vi "test resources list.vi"(8 "error in (no error)":errorcluster) -> (0 "error out":errorcluster, 3 "body":string)   [LabVIEW 2020, in "MCP Server tests.lvlib"]
uses:
  MCP Server tests.lvlib
  <vilib>/JDP Science/JSONtext/Next JSON Value.vi
  <vilib>/JDP Science/JSONtext/String Subset.vi
  <vilib>/JDP Science/JSONtext/Parsing/Advance past next JSON Value (inlined COPY).vi
  <vilib>/JDP Science/JSONtext/Parsing/Advance past whitespace.vi
  <vilib>/JDP Science/JSONtext/Parsing/Advance past String.vi
  <vilib>/JDP Science/JSONtext/Parsing/Advance past Number.vi
  <vilib>/JDP Science/JSONtext/Parsing/Advance past Line Ending.vi
  <vilib>/JDP Science/JSONtext/Parsing/Parse Full Path or Item Name.vi
  <vilib>/JDP Science/JSONtext/Parsing/Advance past Array.vi
  <vilib>/JDP Science/JSONtext/Parsing/Advance past Object.vi
  <vilib>/JDP Science/JSONtext/support/Error Cluster From Code.vi
  <vilib>/JDP Science/JSONtext/Offset/Find Item Locations by Path.vi
  <vilib>/addons/_JKI Toolkits/Caraya/classes/Test/Test.lvclass
  <vilib>/addons/_JKI Toolkits/Caraya/classes/Assert/Assert.lvclass
  <vilib>/JDP Science/JSONtext/JSONtext.lvlib
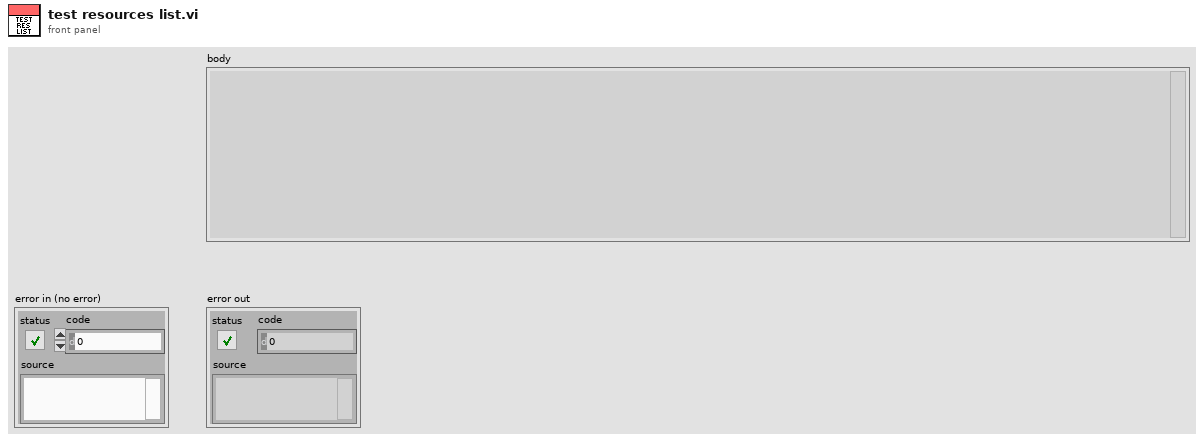
[diagram p1: front panel]
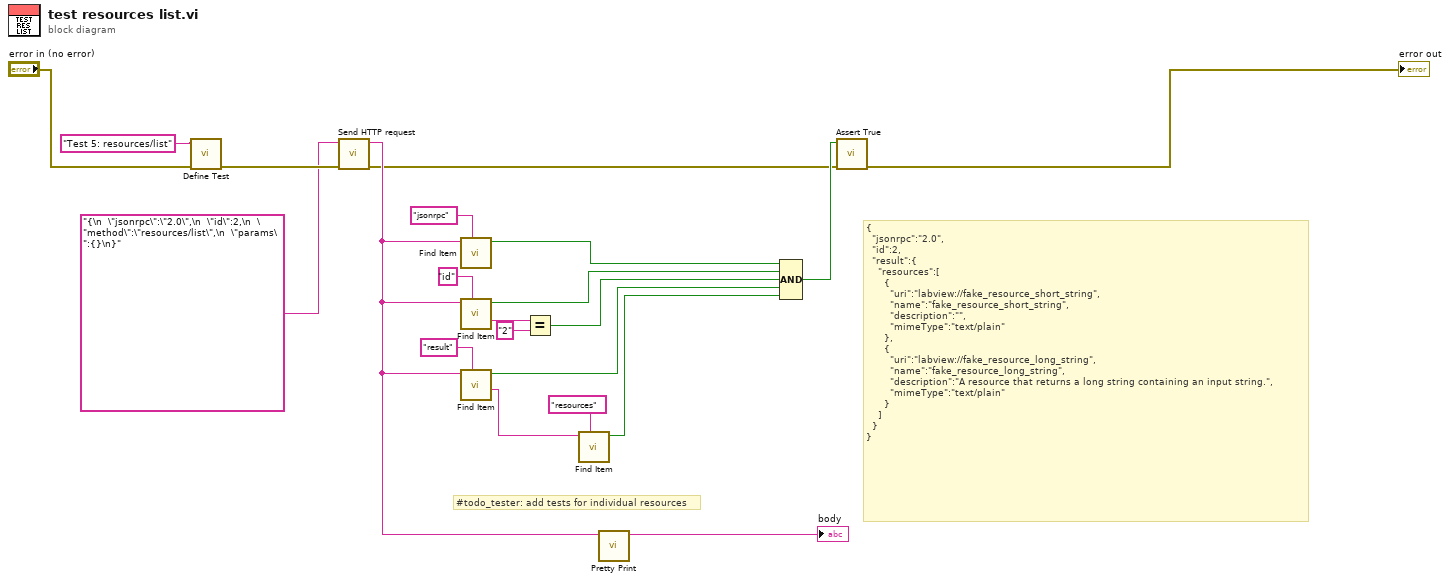
[diagram p0: block diagram]
diagram:
  # "#todo_tester: add tests for individual resources"
  # "{\n  \"jsonrpc\":\"2.0\",\n  \"id\":2,\n  \"result\":{\n    \"resources\":[\n      {\n        \"uri\":\"labview://fake_resource_short_string\",\n        \"name\":\"fake_resource_short_string\",\n        \"description\":\"\",\n        \"mimeType\":\"text/plain\"\n      },\n      {\n        \"uri\":\"labview://fake_resource_long_string\",\n        \"name\":\"fake_resource_long_string\",\n        \"description\":\"A resource that returns a long string containing an input string.\",\n        \"mimeType\":\"text/plain\"\n      }\n    ]\n  }\n}"
  n1 = call <vilib>:"Define Test.vi"("error in (no error)"="error in (no error)", "Label (VI Title)"="Test 5: resources/list") -> ("error out"=w8:errorcluster)  [unwired: 8 in, 1 out]
  n2 = call "Send HTTP request.vi"("error in (no error)"=w8, "request"="{\n  \"jsonrpc\":\"2.0\",\n  \"id\":2,\n  \"method\":\"resources/list\",\n  \"params\":{}\n}" ("buffer")) -> ("error out"=w9:errorcluster, "response"=w20:string)  [unwired: 7 in, 1 out]
  n3 = call <vilib>:"Find Item.vi"("$Path or Item Name"="jsonrpc", "JSON"=w20) -> ("Found"=w14:bool)  [unwired: 6 in, 3 out]
  n4 = call <vilib>:"Find Item.vi"("$Path or Item Name"="id", "JSON"=w20) -> ("<JSON>"=w12:string, "Found"=w15:bool)  [unwired: 6 in, 2 out]
  n5 = call <vilib>:"Find Item.vi"("$Path or Item Name"="result", "JSON"=w20) -> ("<JSON>"=w1:string, "Found"=w19:bool)  [unwired: 6 in, 2 out]
  n6 = Equal?(x=w12, y="2") -> (x = y?=w16:bool)
  n7 = call <vilib>:"Find Item.vi"("$Path or Item Name"="resources", "JSON"=w1) -> ("Found"=w2:bool)  [unwired: 6 in, 3 out]
  n8 = call <vilib>:"Pretty Print.vi"("JSON"=w20) -> ("<JSON>"=→"body":string)  [unwired: 8 in, 2 out]
  n9 = Compound Arithmetic op=AND(w14, w15, w16, w19, w2) -> (w17:bool)
  n10 = call <vilib>:"Assert True.vi"("error in (no error)"=w9, "True?"=w17) -> ("error out"=→"error out":errorcluster)  [unwired: 8 in, 1 out]
